vi "Untitled 4.vi"() -> ()   [LabVIEW 2022 SP3]
uses:
  Control 1.ctl
panel:
  in  "Emp 3":cluster{"Name":string, "Age":dbl}
  in  "Emp 2":cluster{"Name":string, "Age":dbl}
  in  "Emp 1":T1
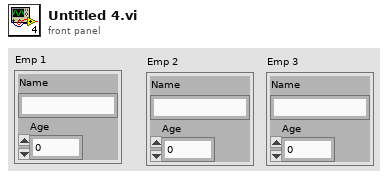
[diagram p1: front panel]
types:
  T1 = typedef "Control 1.ctl" = cluster{"Name":string, "Age":dbl}
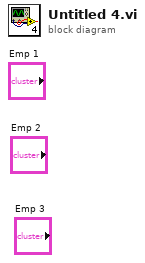
[diagram p0: block diagram]
diagram:
